vi "Write RP EEPROM Calibration.vi"(8 "error in (no error)":errorcluster, 10 "RP EEPROM Calibration":T1, 11 "RP Communicator in":refnum<class "RP Communicator.lvclass">) -> (0 "error out":errorcluster, 3 "RP Communicator out":refnum<class "RP Communicator.lvclass">)   [LabVIEW 2016, in "RP Communicator.lvclass"]
uses:
  RP Communicator.lvclass
  RP EEPROM Calibration.ctl
  RP Communicator.lvclass/RP Communicator.ctl
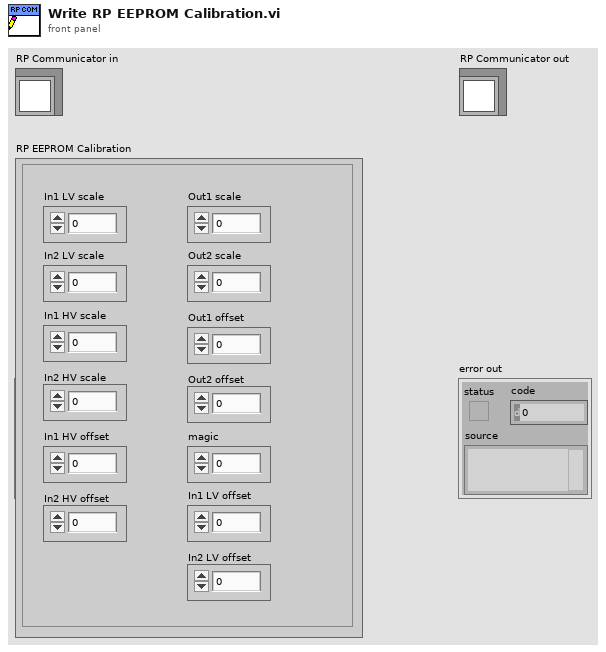
[diagram p1: front panel]
types:
  T1 = typedef "RP EEPROM Calibration.ctl" = cluster{"In1 LV scale":u32, "In2 LV scale":u32, "In1 HV scale":u32, "In2 HV scale":u32, "In1 HV offset":i32, "In2 HV offset":i32, "Out1 scale":u32, "Out2 scale":u32, "Out1 offset":i32, "Out2 offset":i32, "magic":u32, "In1 LV offset":i32, "In2 LV offset":i32}
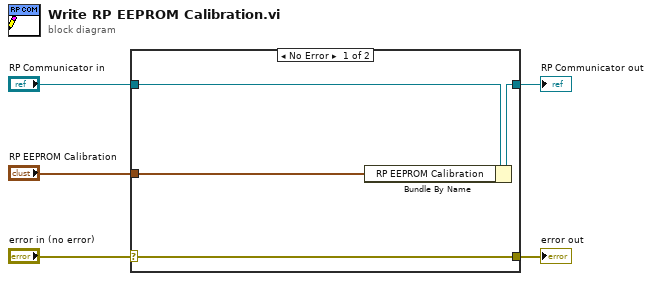
[diagram p0: block diagram]
diagram:
  n1 = case shown="No Error" "error in (no error)" {
    selector: "error in (no error)" -> [w9 w10]
    tunnel: [w9 w10] -> w4
    tunnel: [w7 w11] -> w2
    tunnel: "RP Communicator in" -> [w8 w11]
    tunnel: "RP EEPROM Calibration" -> [w6 _]
    frame No Error {
      n2 = Bundle By Name(cluster=w8, "RP EEPROM Calibration"=w6) -> (w7:refnum<class "RP Communicator.lvclass">)
    }
    frame Error {
    }
  }
  "error out" <- w4
  "RP Communicator out" <- w2
